vi "Gain Scheduling Simulator.vi"() -> ()   [LabVIEW 2023]
doc: "This example demonstrates how to use a gain scheduling PID controller to control a simulated process."
uses:
  <vilib>/addons/control/pid/pid.llb/PID Gain Schedule (DBL).vi
  <vilib>/addons/control/pid/pid.llb/PID (DBL).vi
  <vilib>/addons/control/pid/NI_PID_pid.lvlib
panel:
  out "Output":dbl(graph)
  in  "SP:":dbl(slide)=80.0 min=0.0 max=0.0 scale=0.0..100.0
  out "MV:":dbl(slide)=5.583364480052211 scale=-100.0..100.0
  out "PV:":dbl(slide)=30.663120603565492 scale=0.0..100.0
  out "Plant Variable Lag":dbl=1.4174007085322557
  out "Actual PV":dbl(slide)=30.663120603565492
  out "Plant Variable Gain":dbl=6.132624120713099
  out "Current PID Gains":T1={"proportional gain (Kc)"=100.0, "integral time (Ti, min)"=0.0, "derivative time (Td, min)"=0.0} {"derivative time (Td, min)" format="%.3f"; "integral time (Ti, min)" format="%.3f"; "proportional gain (Kc)" format="%.3f"}
  in  "PID Schedule Parameter":T2(array[cluster])=[{"PID Parameters"={"Kc"=1000.0, "  Ti"=0.0, " Td"=0.0}, "Max PV"=0.0}, {"PID Parameters"={"Kc"=500.0, "  Ti"=0.0, " Td"=0.0}, "Max PV"=20.0}, {"PID Parameters"={"Kc"=100.0, "  Ti"=0.0, " Td"=0.0}, "Max PV"=40.0}, {"PID Parameters"={"Kc"=50.0, "  Ti"=0.01, " Td"=0.0}, "Max PV"=60.0}, {"PID Parameters"={"Kc"=10.0, "  Ti"=0.05, " Td"=0.0}, "Max PV"=80.0}, {"PID Parameters"={"Kc"=5.0, "  Ti"=0.05, " Td"=0.001}, "Max PV"=100.0}] {"Max PV" format="%#.2f"; "PID Parameters"."Td" format="%#.3g"; "PID Parameters"."Ti" format="%#.3g"; "PID Parameters"."Kc" format="%#.3f"}
  in  "Stop":bool
  out "Process Variable/Setpoint/Output":cluster{"Plant Output":dbl, "SP1:":dbl}(graph)
  # "Overview: This example demonstrates how to use a gain scheduling PID controller to control a simulated process.\nInstructions:\n1. Run the VI and observe the Current PID Gains being changed according to the value of the PV.\n2. Click Stop to stop the VI."
  # "PID"
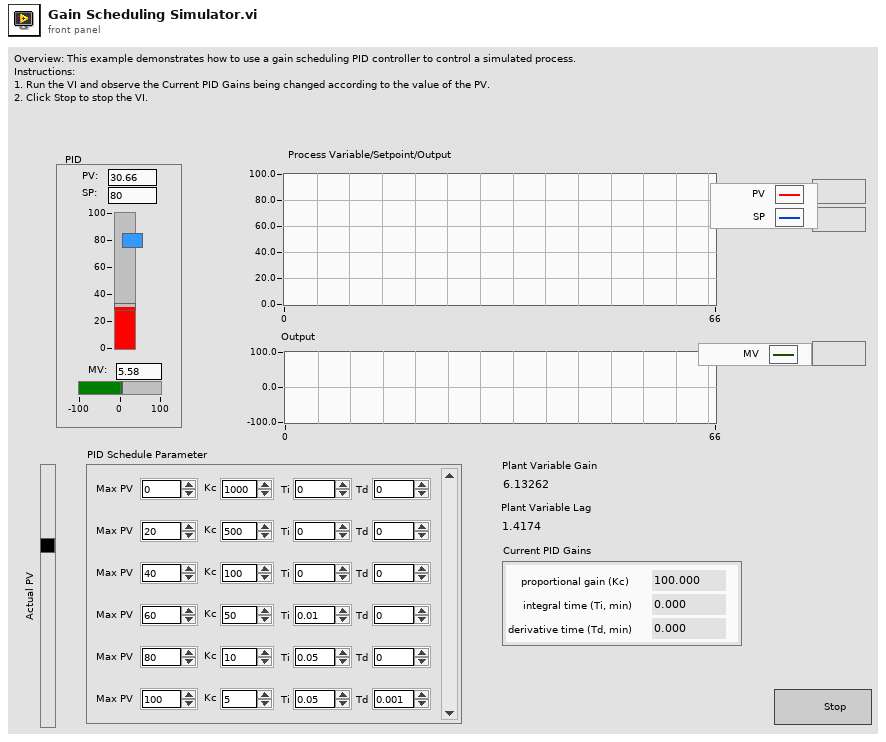
[diagram p1: front panel]
types:
  T1 = cluster{"proportional gain (Kc)":dbl, "integral time (Ti, min)":dbl, "derivative time (Td, min)":dbl}
  T2 = cluster{"PID Parameters":cluster{"Kc":dbl, "  Ti":dbl, " Td":dbl}, "Max PV":dbl}[]
  T3 = cluster{"static gain":dbl, "lag (min)":dbl, "dead cycles":dbl, "load %":dbl, "deadband":dbl, "noise level %":dbl, "initial PV":dbl, "initial PV 2":dbl}
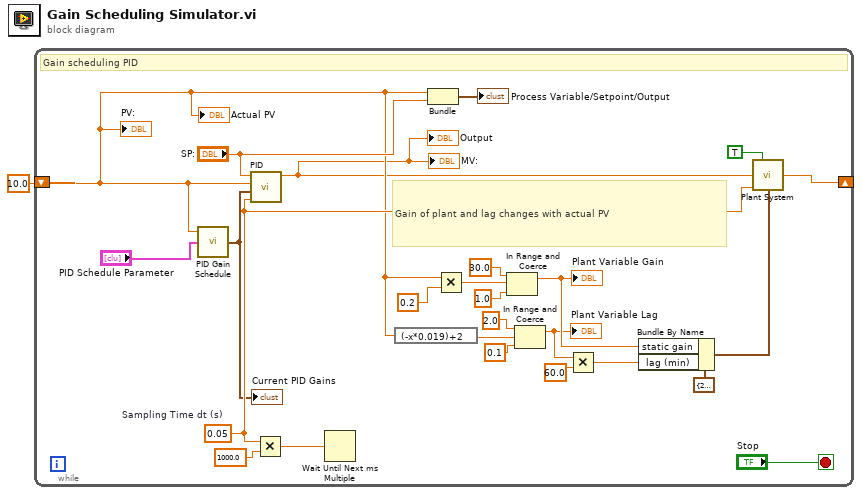
[diagram p0: block diagram]
diagram:
  n1 = while {
    shift-left: 10.0 ("Plant Output") -> [w12]
    shift-right: [w24] -> _
    stop <- "Stop" stop-if-true
    w22 = 0.05  # Sampling Time dt (s)
    # "Gain of plant and lag changes with actual PV"
    # "Gain scheduling PID"
    n2 = call-poly <vilib>:"PID Gain Schedule.vi"("PID gain schedule"="PID Schedule Parameter", "gain scheduling value"=w12) -> ("PID gains out"=w16:T1)  [unwired: 2 in, 1 out]
    "Current PID Gains" <- w16
    n3 = call-poly <vilib>:"PID.vi"("dt (s)"=w22, "PID gains"=w16, "process variable"=w12, "setpoint"="SP:") -> ("output"=w4:dbl)  [unwired: 6 in, 1 out]
    "MV:" <- w4
    "Output" <- w4
    n4 = Multiply(x=w22, y=1000.0) -> (x*y=w3:dbl)
    n5 = Wait Until Next ms Multiple(millisecond multiple=w3) -> ()  [unwired: 1 out]
    n6 = expression code="(-x*0.019)+2"(w12) -> (w11:dbl)
    n7 = Bundle("Plant Output"=w12, "SP:"="SP:") -> (→"Process Variable/Setpoint/Output":cluster{"Plant Output":dbl, "SP:":dbl})  [unwired: 1 in]
    n8 = Multiply(x=w12, y=0.2) -> (x*y=w17:dbl)
    n9 = In Range and Coerce(upper limit=30.0, x=w17, lower limit=1.0) -> (coerced(x)=w10:dbl)  [unwired: 1 out]
    "Plant Variable Gain" <- w10
    n10 = In Range and Coerce(upper limit=2.0, x=w11, lower limit=0.1) -> (coerced(x)=w9:dbl)  [unwired: 1 out]
    "Plant Variable Lag" <- w9
    n11 = Multiply(x=w9, y=60.0 ("x")) -> (x*y=w7:dbl)
    n12 = Bundle By Name(cluster=T3 {"static gain"=2.5, "lag (min)"=18.0, "dead cycles"=0.0, "load %"=40.0, "deadband"=2.0, "noise level %"=0.25, "initial PV"=10.0, "initial PV 2"=0.0} ("process parameters"), "static gain"=w10, "lag (min)"=w7) -> (w8:T3)
    n13 = call "Plant System.vi"("Integrator ?"=TRUE, "Plant Input"=w4, "dt (s)"=w22, "process parameters"=w8) -> ("Plant Output"=w24:dbl)  [unwired: 11 in]
    "PV:" <- w12
    "Actual PV" <- w12
  }
